vi "MC_README.vi"   [LabVIEW 2009]
uses:
  SRV VIs/SubVIs/SRVGlobals.vi
panel:
  # "MC\nREADME"
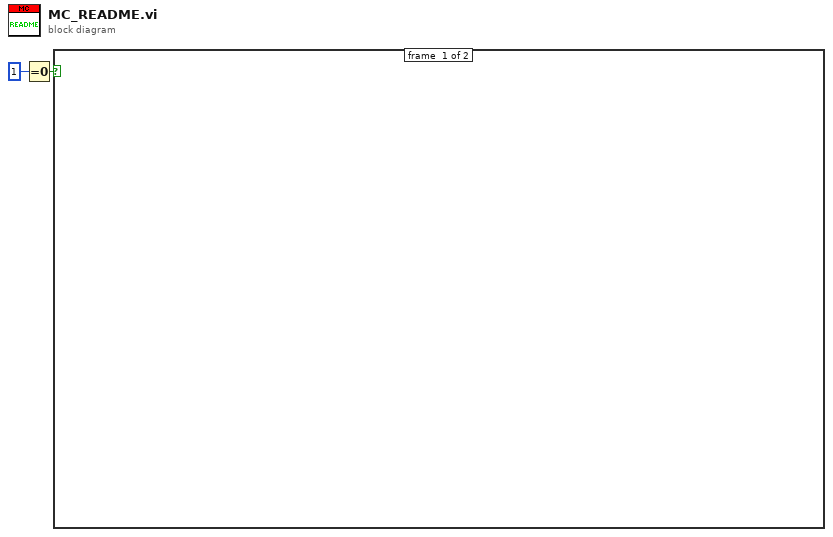
[diagram p0: block diagram]
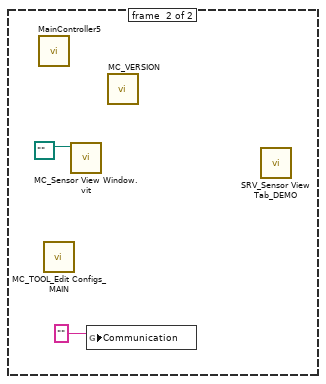
[diagram p2: hidden frame]
diagram:
  n1 = Equal To 0?(x=1) -> (x = 0?=w1:bool)
  n2 = case shown="True" w1 {
    frame #0 {
    }
    frame #1 {
      n3 = call "MainController5.vi"() -> ()  [unwired: 1 in]
      n4 = call "MC_TOOL_Edit Configs_MAIN.vi"() -> ()  [unwired: 11 in, 1 out]
      n5 = call "MC_Sensor View Window.vit"("Sensors Config File Path"=path "") -> ()  [unwired: 10 in, 1 out]
      n6 = global write "SRVGlobals.vi" "Communication"("" ("Communication")) -> ()
      n7 = call "MC_VERSION.vi"() -> ()  [unwired: 1 out]
      n8 = call "SRV_Sensor View Tab_DEMO.vi"() -> ()  [unwired: 1 in]
    }
  }
